vi "__Cleanup.vi"(8 "error in (no error)":errorcluster, 11 "FileManager Data in":T1) -> (0 "error out":errorcluster)   [LabVIEW 2011]
doc: "This VI clears data from the ComboBoxes and ListBoxes, and closes their references."
uses:
  __File manager Data type.ctl
  <vilib>/Utility/miscctls.llb/LVRowAndColumnUnsignedTypeDef.ctl
  <vilib>/Utility/miscctls.llb/LVComboBoxStrsAndValuesArrayTypeDef.ctl
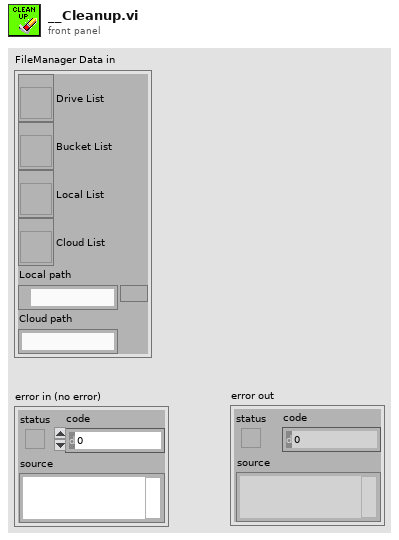
[diagram p1: front panel]
types:
  T1 = typedef "__File manager Data type.ctl" = cluster{"Drive List":refnum<vi>, "Bucket List":refnum<vi>, "Local List":refnum<vi>, "Cloud List":refnum<vi>, "Local path":path, "Cloud path":string}
  T2 = typedef "LVRowAndColumnUnsignedTypeDef.ctl" = cluster{"Row":u32, "Column":u32}
  T3 = typedef "LVComboBoxStrsAndValuesArrayTypeDef.ctl" = cluster{"String":string, "Value":string}[]
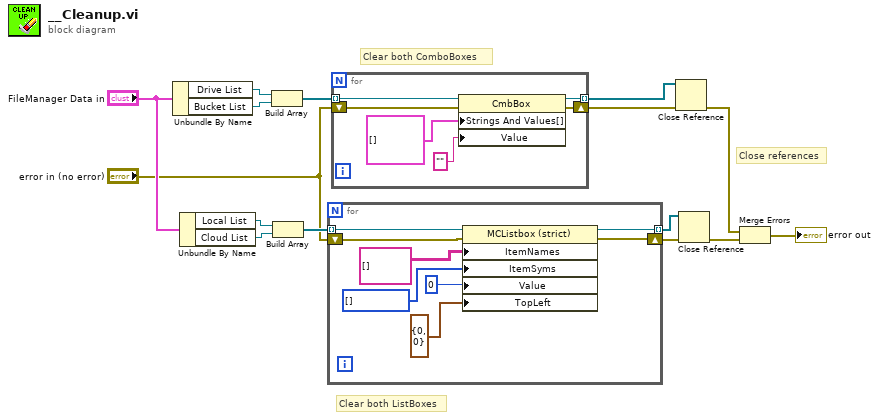
[diagram p0: block diagram]
diagram:
  # "Close references"
  # "Clear both ListBoxes"
  # "Clear both ComboBoxes"
  n1 = Unbundle By Name("FileManager Data in") -> ("Drive List"=w15:refnum<vi>, "Bucket List"=w14:refnum<vi>)
  n2 = Unbundle By Name("FileManager Data in") -> ("Local List"=w9:refnum<vi>, "Cloud List"=w8:refnum<vi>)
  n3 = Build Array(w15, w14) -> (w13:refnum<vi>[])
  n4 = Build Array(w9, w8) -> (w7:refnum<vi>[])
  n5 = for {
    tunnel: w7 -> [w19] mode=indexing
    shift-right: [w17] -> w5
    shift-left: "error in (no error)" -> [w18]
    tunnel: [w16] -> w4 mode=indexing
    n6 = property class="MCListbox (strict)"(reference=w19, error in=w18, "ItemNames"=string[][] [], "ItemSyms"=i32[] [], "Value"=0, "TopLeft"=T2 {"Row"=0, "Column"=0} ("Top Left Visible Cell")) -> (reference out=w16:refnum<vi>, error out=w17:errorcluster)
  }
  n7 = for {
    tunnel: w13 -> [w29] mode=indexing
    shift-right: [w26] -> w12
    shift-left: "error in (no error)" -> [w27]
    tunnel: [w25] -> w11 mode=indexing
    n8 = property class="CmbBox"(reference=w29, error in=w27, "Strings And Values[]"=T3 [] ("Strings And Values []"), "Value"="") -> (reference out=w25:refnum<vi>, error out=w26:errorcluster)
  }
  n9 = Close Reference(reference=w11, error in (no error)=w12) -> (error out=w2:errorcluster)
  n10 = Close Reference(reference=w4, error in (no error)=w5) -> (error out=w3:errorcluster)
  n11 = Merge Errors(w2, w3) -> (→"error out":errorcluster)
